vi "Live window-Snapshot handler.vi"(6 "Window ctrl refs":T1, 9 "Right image":T3, 10 "Left image":T3, 11 "Snapshot:NewVal":bool) -> ()   [LabVIEW 2017]
uses:
  <vilib>/vision/Image Controls.llb/IMAQ Image.ctl
  Typedefs/Live window-ctrl refs.ctl
  Typedefs/Channel Selector.ctl
  Typedefs/Image display ref.ctl
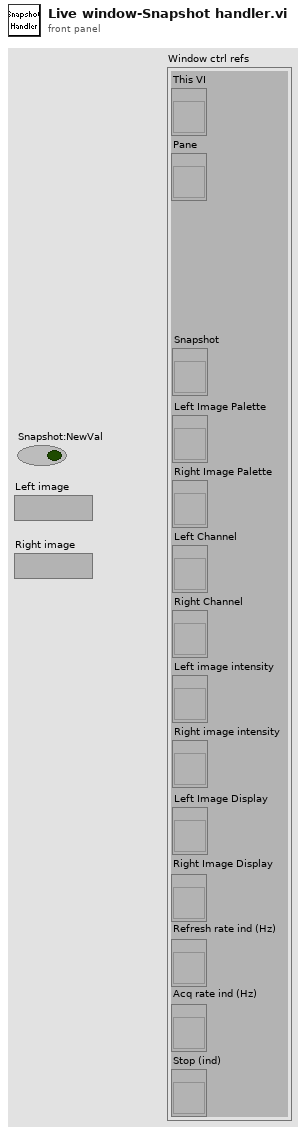
[diagram p1: front panel]
types:
  T1 = typedef "Live window-ctrl refs.ctl" = cluster{"This VI":refnum<vi>, "Pane":refnum<vi>, "Snapshot":refnum<vi>, "Left Image Palette":refnum<vi>, "Right Image Palette":refnum<vi>, "Left Channel":refnum<vi>, "Right Channel":refnum<vi>, "Left image intensity":refnum<vi>, "Right image intensity":refnum<vi>, "Left Image Display":T2, "Right Image Display":T2, "Refresh rate ind (Hz)":refnum<vi>, "Acq rate ind (Hz)":refnum<vi>, "Stop (ind)":refnum<vi>}
  T2 = typedef "Image display ref.ctl" = refnum<vi>
  T3 = typedef "IMAQ Image.ctl" = refnum<image>
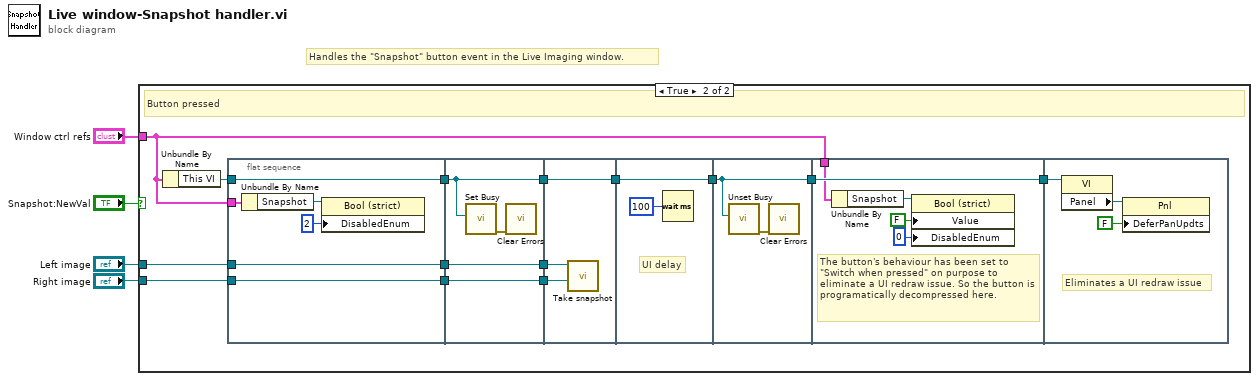
[diagram p0: block diagram]
diagram:
  # "Handles the \"Snapshot\" button event in the Live Imaging window."
  n1 = case shown="True" "Snapshot:NewVal" {
    tunnel: "Left image" -> [_ w14]
    tunnel: "Right image" -> [_ w12]
    tunnel: "Window ctrl refs" -> [_ w5]
    frame False {
      # "Button released"
    }
    frame True {
      # "Button pressed"
      n2 = Unbundle By Name(w5) -> ("This VI"=w18:refnum<vi>)
      n3 = flat-sequence {
        tunnel: w12 -> [w22]
        tunnel: w14 -> [w23]
        tunnel: w18 -> [w24]
        tunnel: [w24] -> w10
        tunnel: [w23] -> w9
        tunnel: [w22] -> w8
        tunnel: w5 -> [w19]
        tunnel: [w27] -> w15
        tunnel: [w26] -> w13
        tunnel: [w25] -> w11
        tunnel: w10 -> [w27]
        tunnel: w9 -> [w26]
        tunnel: w8 -> [w25]
        tunnel: [w31] -> w16
        tunnel: w15 -> [w31]
        tunnel: w13 -> [w30]
        tunnel: w11 -> [w29]
        tunnel: [w32] -> w17
        tunnel: w16 -> [w32]
        tunnel: w17 -> [w34]
        tunnel: [w34] -> w7
        tunnel: w7 -> [w40]
        tunnel: [w40] -> w6
        tunnel: w5 -> [w36]
        tunnel: w6 -> [w41]
        frame #0 {
          n4 = Unbundle By Name(w19) -> ("Snapshot"=w21:refnum<vi>)
          n5 = property class="Bool (strict)"(reference=w21, "DisabledEnum"=2) -> ()  [unwired: 1 in, 2 out]
        }
        frame #1 {
          n6 = call <vilib>:"Set Busy.vi"("VI reference (current VI)"=w27) -> ("error out"=w28:errorcluster)  [unwired: 9 in, 1 out]
          n7 = call <vilib>:"Clear Errors.vi"("error in (no error)"=w28) -> ()  [unwired: 5 in, 2 out]
        }
        frame #2 {
          n8 = call "Take snapshot.vi"("Right Image"=w29, "Left Image"=w30) -> ()  [unwired: 10 in]
        }
        frame #3 {
          # "UI delay"
          n9 = Wait (ms)(milliseconds to wait=u32 100) -> ()  [unwired: 1 out]
        }
        frame #4 {
          n10 = call <vilib>:"Unset Busy.vi"("VI reference (current VI)"=w34) -> ("error out"=w35:errorcluster)  [unwired: 10 in]
          n11 = call <vilib>:"Clear Errors.vi"("error in (no error)"=w35) -> ()  [unwired: 5 in, 2 out]
        }
        frame #5 {
          # "The button's behaviour has been set to \"Switch when pressed\" on purpose to eliminate a UI redraw issue. So the button is programatically decompressed here."
          n12 = Unbundle By Name(w36) -> ("Snapshot"=w38:refnum<vi>)
          n13 = property class="Bool (strict)"(reference=w38, "Value"=FALSE ("Snapshot"), "DisabledEnum"=0) -> ()  [unwired: 1 in, 2 out]
        }
        frame #6 {
          # "Eliminates a UI redraw issue"
          n14 = property class="VI"(reference=w41) -> ("Panel"=w42:refnum<vi>)  [unwired: 1 in, 2 out]
          n15 = property class="Pnl"(reference=w42, "DeferPanUpdts"=FALSE ("Defer Panel Updates")) -> ()  [unwired: 1 in, 2 out]
        }
      }
    }
  }
